vi "Program01 (b).vi"() -> ()   [LabVIEW 2015]
uses:
  <vilib>/measure/NI_MABase.lvlib
panel:
  in  "sampling info":cluster{"Fs":dbl, "#s":dbl}={"Fs"=1000.0, "#s"=1000.0} {"Fs" format="%.2p"}
  in  "seed":i32=-1
  in  "amplitude 2":dbl=1.0 format="%.2p"
  out "demodulated signal":dynamicdata(graph)=[{"t0"=timestamp(0 s since 1904-01-01), "dt"=0.0003333333333333333, "Y"=array[1000 elements], "attributes"=variant("NI_ChannelName"=variant(string "Filtered"))}]
  out "Modulated signal":dynamicdata(graph)
  in  "sampling info 2":cluster{"Fs":dbl, "#s":dbl}={"Fs"=3000.0, "#s"=1000.0} {"Fs" format="%.2p"}
  out "Carrier signal":waveform(dbl)(graph)={"t0"=timestamp(0 s since 1904-01-01), "dt"=0.0003333333333333333, "Y"=array[1000 elements]}
  out "Modulating signal":dynamicdata(graph)
  in  "signal type":T1(ring)
  in  "phase":dbl format="%.2p"
  in  "amplitude":dbl=1.0 format="%0.2p"
  in  "frequency":dbl=10.0 format="%0.2p"
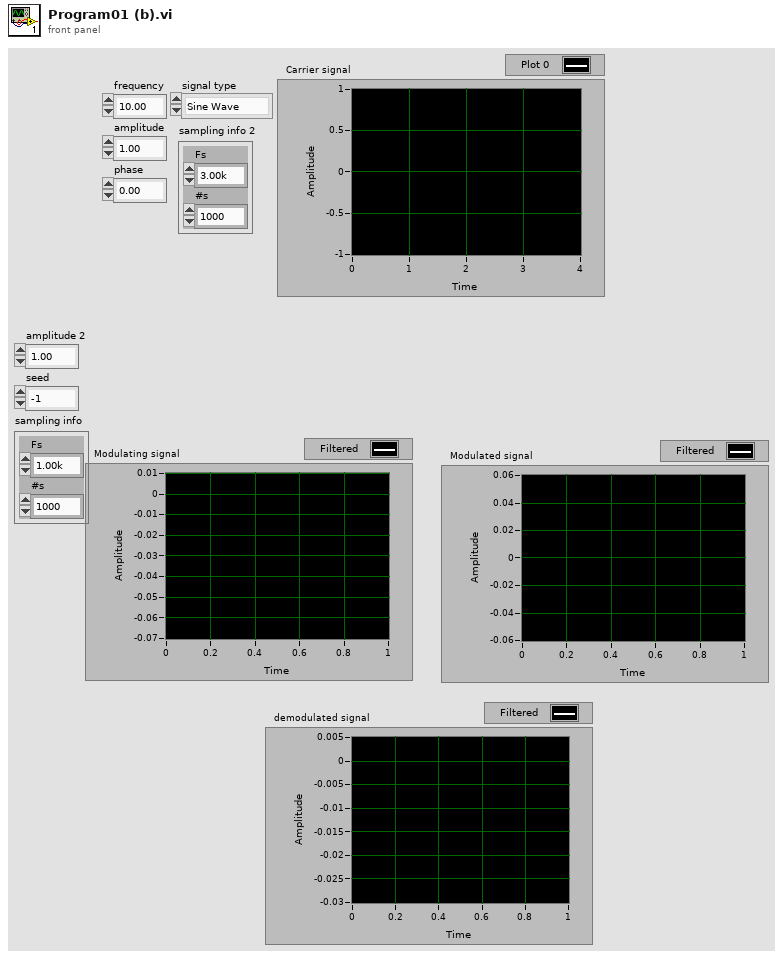
[diagram p1: front panel]
types:
  T1 = enum16{"Sine Wave", "Triangle Wave", "Square Wave", "Sawtooth Wave"}
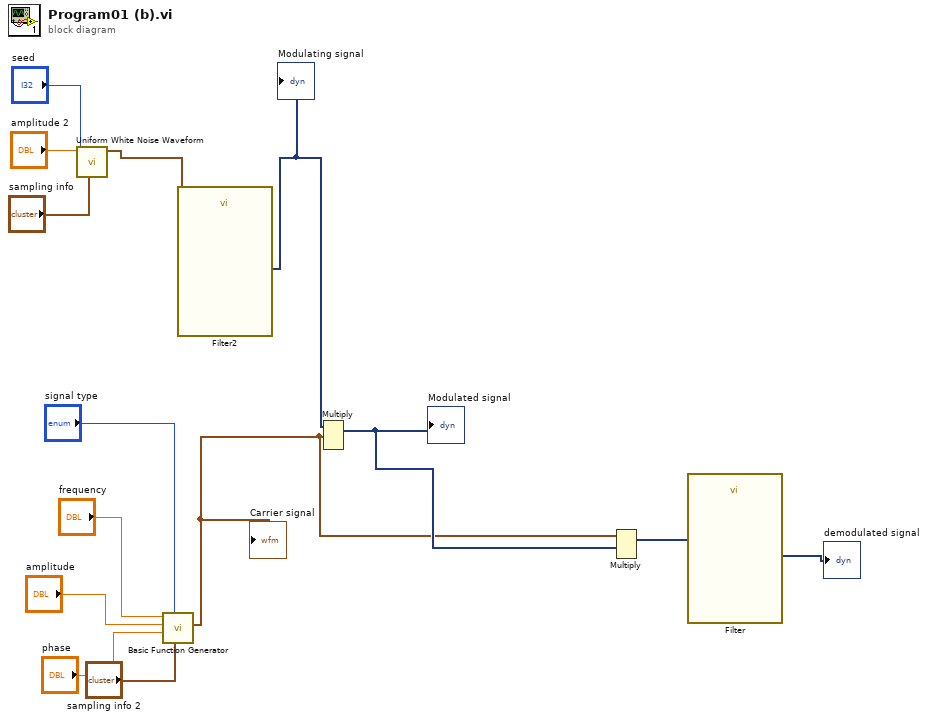
[diagram p0: block diagram]
diagram:
  n1 = call <vilib>:"Uniform White Noise Waveform.vi"("sampling info"="sampling info", "seed"="seed", "amplitude"="amplitude 2") -> ("signal out"=w3:waveform(dbl))  [unwired: 7 in, 1 out]
  n2 = call <vilib>:"Basic Function Generator.vi"("sampling info"="sampling info 2", "signal type"="signal type", "phase"="phase", "amplitude"="amplitude", "frequency"="frequency") -> ("signal out"=w1:waveform(dbl))  [unwired: 4 in, 2 out]
  "Carrier signal" <- w1
  n3 = call "Filter2"("Signal"=w3) -> ("Filtered Signal"=w2:dynamicdata)  [unwired: 9 in, 1 out]
  "Modulating signal" <- w2
  n4 = Multiply(1:w1, 2:w2) -> (0:w8:dynamicdata)  [unwired: 1 in, 1 out]
  "Modulated signal" <- w8
  n5 = Multiply(1:w8, 2:w1) -> (0:w9:dynamicdata)  [unwired: 1 in, 1 out]
  n6 = call "Filter"("Signal"=w9) -> ("Filtered Signal"=→"demodulated signal":dynamicdata)  [unwired: 9 in, 1 out]
